vi "somethingelseIcantremember.vi"(11 "GObject in":refnum<vi>) -> (3 "Colors [4]":cluster{u32, u32}[](array[cluster]))   [LabVIEW 2014]
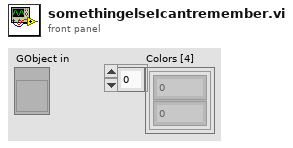
[diagram p1: front panel]
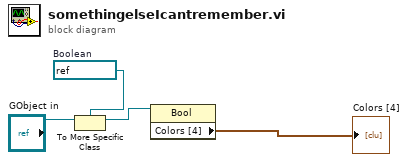
[diagram p0: block diagram]
diagram:
  w2 = refnum<vi> refnum  # Boolean
  n1 = To More Specific Class(target class=w2, reference="GObject in") -> (specific class reference=w3:refnum<vi>)  [unwired: 1 in, 1 out]
  n2 = property class="Bool"(reference=w3) -> ("Colors [4]"=→"Colors [4]":cluster{u32, u32}[])  [unwired: 1 in, 2 out]
